vi "GetTimingInfo.vi"() -> (1 "TimingInfo":string[](array[string]), 2 "Error":bool)   [LabVIEW 2014]
panel:
  out "TimingMaximums":string[](array[string])
  out "TimingMinimums":string[](array[string])
  out "TimingValues":string[](array[string])
  out "TimingNames":string[](array[string])
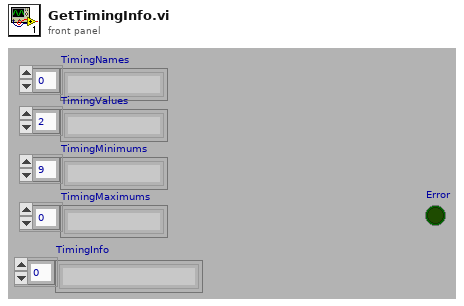
[diagram p1: front panel]
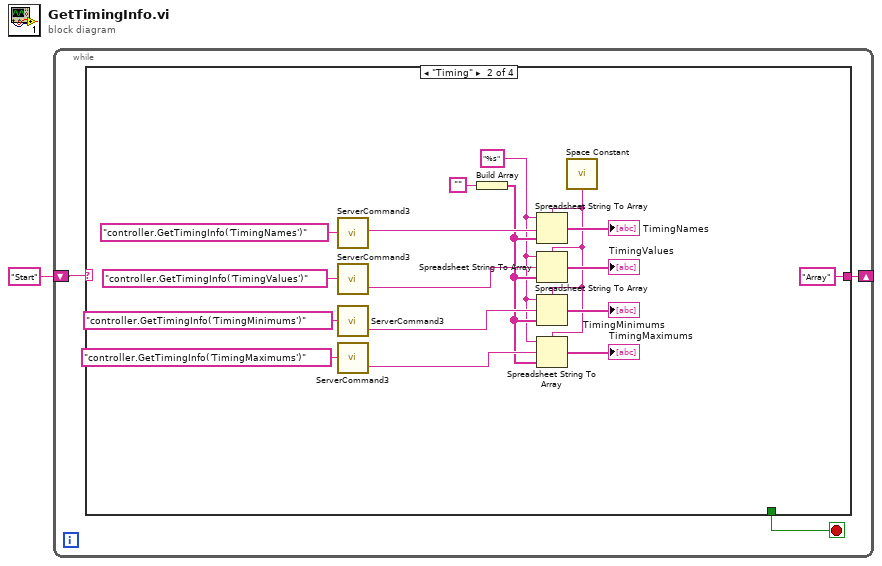
[diagram p0: block diagram]
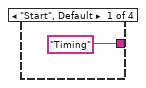
[diagram p2: hidden frame]
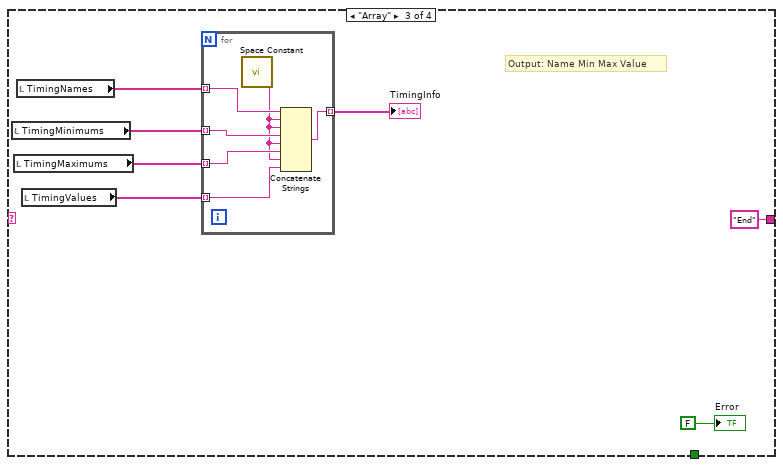
[diagram p3: hidden frame]
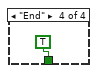
[diagram p4: hidden frame]
diagram:
  n1 = while {
    shift-right: [w4] -> _
    shift-left: "Start" ("Command") -> [w3]
    stop <- w2 stop-if-true
    n2 = case shown="\"Timing\"" w3 {
      tunnel: ["Timing" ("Command") "Array" ("Command") "End" ("Command") _] -> w4
      tunnel: [_ _ _ TRUE] -> w2
      frame "Start", Default {
      }
      frame "Timing" {
        w7 = "%s" ("format string")
        n3 = call "ServerCommand3.vi"("Command"="controller.GetTimingInfo('TimingNames')") -> ("Reply"=w12:string)  [unwired: 1 out]
        n4 = call "ServerCommand3.vi"("Command"="controller.GetTimingInfo('TimingValues')") -> ("Reply"=w11:string)  [unwired: 1 out]
        n5 = call "ServerCommand3.vi"("Command"="controller.GetTimingInfo('TimingMinimums')") -> ("Reply"=w10:string)  [unwired: 1 out]
        n6 = call "ServerCommand3.vi"("Command"="controller.GetTimingInfo('TimingMaximums')") -> ("Reply"=w9:string)  [unwired: 1 out]
        n7 = Build Array("") -> (w8:string[])
        n8 = call <vilib>:"Space Constant.vi"() -> ("String"=w6:string)
        n9 = Spreadsheet String To Array(delimiter (Tab)=w6, format string=w7, spreadsheet string=w12, array type (2D Dbl)=w8) -> (array=→"TimingNames":string[])
        n10 = Spreadsheet String To Array(delimiter (Tab)=w6, format string=w7, spreadsheet string=w11, array type (2D Dbl)=w8) -> (array=→"TimingValues":string[])
        n11 = Spreadsheet String To Array(delimiter (Tab)=w6, format string=w7, spreadsheet string=w10, array type (2D Dbl)=w8) -> (array=→"TimingMinimums":string[])
        n12 = Spreadsheet String To Array(delimiter (Tab)=w6, format string=w7, spreadsheet string=w9, array type (2D Dbl)=w8) -> (array=→"TimingMaximums":string[])
      }
      frame "Array" {
        # "Output: Name Min Max Value"
        n13 = local read "TimingMinimums"() -> (w27:string[])
        n14 = local read "TimingMaximums"() -> (w26:string[])
        n15 = local read "TimingNames"() -> (w28:string[])
        n16 = local read "TimingValues"() -> (w25:string[])
        n17 = for {
          tunnel: w28 -> [w31] mode=indexing
          tunnel: w27 -> [w35] mode=indexing
          tunnel: w26 -> [w34] mode=indexing
          tunnel: w25 -> [w33] mode=indexing
          tunnel: [w32] -> w23 mode=indexing
          n18 = call <vilib>:"Space Constant.vi"() -> ("String"=w30:string)
          n19 = Concatenate Strings(w31, w30, w30, w35, w30, w34, w30, w33) -> (w32:string)
        }
        "TimingInfo" <- w23
        "Error" <- FALSE ("Error")
      }
      frame "End" {
      }
    }
  }
